vi "buttonsexample.vi"() -> ()   [LabVIEW 2015]
panel:
  in  "Numeric":i32
  in  "stop":bool
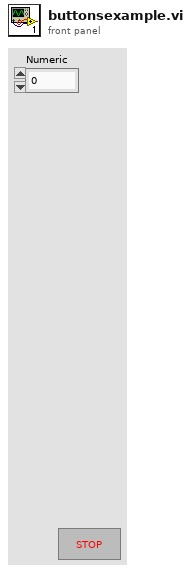
[diagram p1: front panel]
types:
  T1 = enum16{"Left Button", "Center Button", "Right Button", "Window Close"}
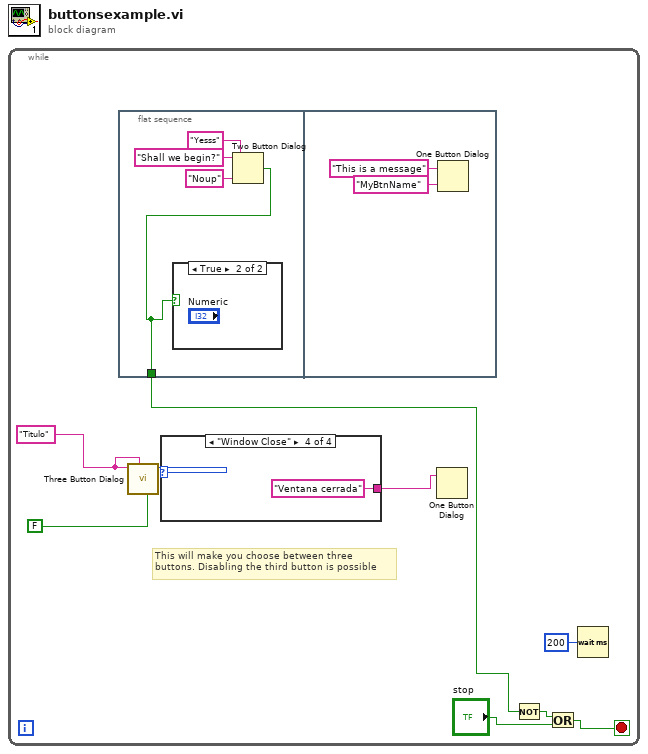
[diagram p0: block diagram]
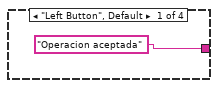
[diagram p2: hidden frame]
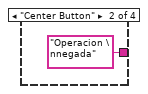
[diagram p3: hidden frame]
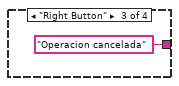
[diagram p4: hidden frame]
diagram:
  n1 = while {
    stop <- w1 stop-if-true
    w8 = "Titulo" ("message")
    # "This will make you choose between three\nbuttons. Disabling the third button is possible"
    n2 = flat-sequence {
      tunnel: [w14] -> w2
      frame #0 {
        n3 = Two Button Dialog(message="Shall we begin?", 1:"Noup" ("F button name (\"Cancel\")"), 2:"Yesss" ("T button name (\"OK\")")) -> (T button?=w14:bool)
        n4 = case shown="True" w14 {
          frame False {
          }
          frame True {
          }
        }
      }
      frame #1 {
        n5 = One Button Dialog(message="This is a message", button name ("OK")="MyBtnName") -> ()  [unwired: 1 out]
      }
    }
    n6 = call <vilib>:"Three Button Dialog.vi"("Allow user to close window? (TRUE)"=FALSE, "Window Title (\"\")"=w8, "message"=w8) -> ("Which Button?"=w7:T1)  [unwired: 8 in]
    n7 = case shown="\"Window Close\"" w7 {
      tunnel: ["Operacion aceptada" "Operacion \nnegada" "Operacion cancelada" "Ventana cerrada"] -> w6
      frame "Left Button", Default {
      }
      frame "Center Button" {
      }
      frame "Right Button" {
      }
      frame "Window Close" {
      }
    }
    n8 = One Button Dialog(message=w6) -> ()  [unwired: 1 in, 1 out]
    n9 = Not(x=w2) -> (.not. x?=w3:bool)
    n10 = Or(x=w3, y="stop") -> (x .or. y?=w1:bool)
    n11 = Wait (ms)(milliseconds to wait=u32 200) -> ()  [unwired: 1 out]
  }
